vi "S2C_Shared_Proc_CommandCheck.vi"(7 "Cmd In":string) -> (2 "Local?":bool, 8 "Cmd Out":string)   [LabVIEW 2024]
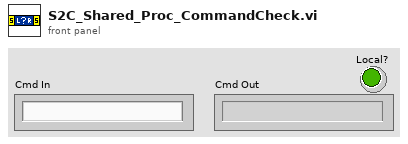
[diagram p1: front panel]
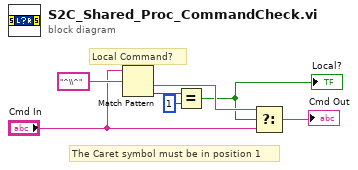
[diagram p0: block diagram]
diagram:
  # "The Caret symbol must be in position 1"
  # "Local Command?"
  n1 = Match Pattern(string="Cmd In", regular expression="^\\^") -> (after substring=w4:string, offset past match=w6:i32)  [unwired: 1 in, 2 out]
  n2 = Equal?(x=w6, y=1) -> (x = y?=w1:bool)
  "Local?" <- w1
  n3 = Select(t=w4, s=w1, f="Cmd In") -> (s? t:f=→"Cmd Out":string)
